vi "Write Increment.vi"(8 "error in (no error)":errorcluster, 10 "Increment":i32, 11 "Counter Config in":refnum<class "Counter Config.lvclass">) -> (0 "error out":errorcluster, 3 "Counter Config out":refnum<class "Counter Config.lvclass">)   [LabVIEW 2015, in "Counter Config.lvclass"]
uses:
  Counter Config.lvclass
  Counter Config.lvclass/Counter Config.ctl
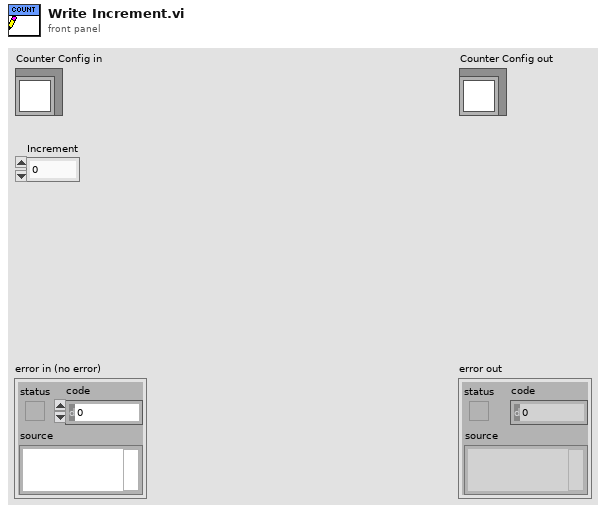
[diagram p1: front panel]
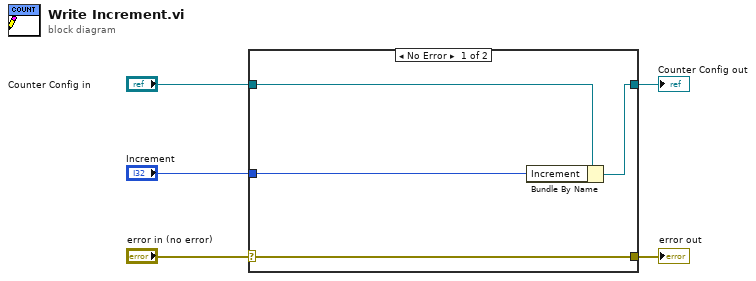
[diagram p0: block diagram]
diagram:
  n1 = case shown="No Error" "error in (no error)" {
    selector: "error in (no error)" -> [w9 w10]
    tunnel: [w9 w10] -> w4
    tunnel: [w7 w11] -> w2
    tunnel: "Counter Config in" -> [w8 w11]
    tunnel: "Increment" -> [w6 _]
    frame No Error {
      n2 = Bundle By Name(cluster=w8, "Increment"=w6) -> (w7:refnum<class "Counter Config.lvclass">)
    }
    frame Error {
    }
  }
  "error out" <- w4
  "Counter Config out" <- w2
